vi "Close.vi"(8 "error in (no error)":errorcluster, 11 "Driver in":refnum<class "Driver.lvclass">) -> (0 "error out":errorcluster, 3 "Driver out":refnum<class "Driver.lvclass">)   [LabVIEW 2023, in "Driver.lvlib" / "Driver.lvclass"]
uses:
  Driver.lvclass
  Driver.lvclass/Driver.ctl
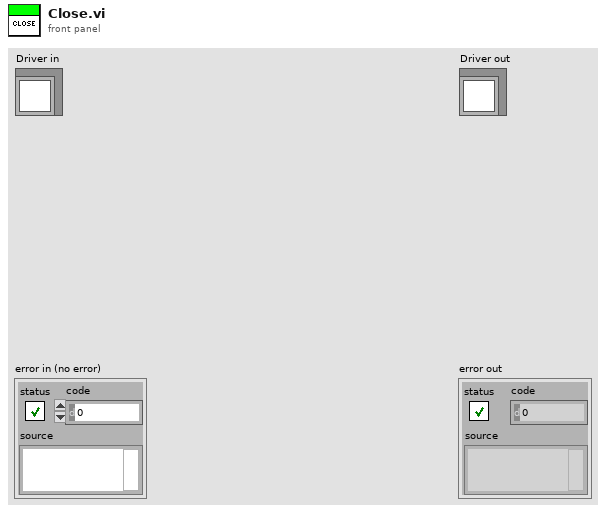
[diagram p1: front panel]
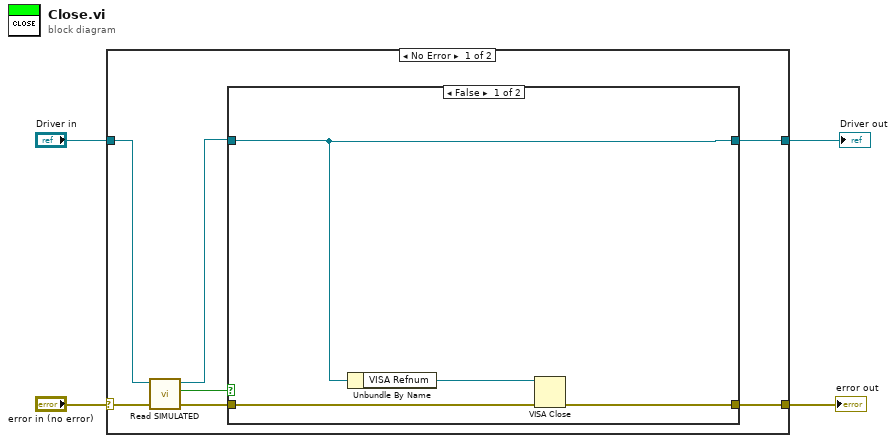
[diagram p0: block diagram]
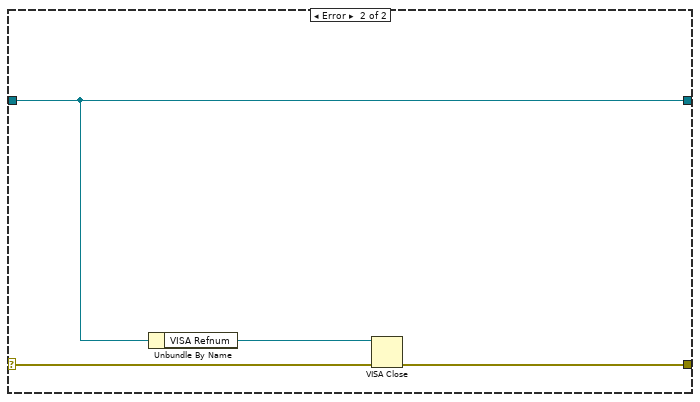
[diagram p3: hidden frame]
diagram:
  n1 = case shown="No Error" "error in (no error)" {
    selector: "error in (no error)" -> [w8 w21]
    tunnel: [w11 w20] -> w3
    tunnel: "Driver in" -> [w10 w19]
    tunnel: [w5 w19] -> w1
    frame No Error {
      n2 = call-dynamic "Read SIMULATED.vi"("error in (no error)"=w8, "Driver in"=w10) -> ("error out"=w7:errorcluster, "SIMULATED"=w6:bool, "Driver out"=w9:refnum<class "Driver.lvclass">)  [unwired: 7 in]
      n3 = case shown="False" w6 {
        tunnel: w7 -> [w15 w16]
        tunnel: [w14 w16] -> w11
        tunnel: w9 -> [w12 w17]
        tunnel: [w12 w17] -> w5
        frame False {
          n4 = Unbundle By Name(w12) -> ("VISA Refnum"=w13:refnum<visa-resource-name>)
          n5 = VISA Close(VISA resource name=w13, error in (no error)=w15) -> (error out=w14:errorcluster)
        }
        frame True {
        }
      }
    }
    frame Error {
      n6 = Unbundle By Name(w19) -> ("VISA Refnum"=w18:refnum<visa-resource-name>)
      n7 = VISA Close(VISA resource name=w18, error in (no error)=w21) -> (error out=w20:errorcluster)
    }
  }
  "error out" <- w3
  "Driver out" <- w1
